vi "CTRE_Phoenix_MotorControl_PushMotionProfileTrajectory.vi"(0 "PhoenixMotorControlDevRef":T2={"DeviceStatus"={"status"=FALSE, "code"=0, "source"=""}, "Type"=enum."PWM", "PWM"={"PWM Channel"=enum."Invalid", "DeadBand"={"Name"="", "maxPositivePwm"=0, "minPositivePwm"=0, "centerPwm"=0, "maxNegativePwm"=0, "minNegativePwm"=0, "angularRange"=0}}, "CAN"={"Device Number"=0, "SetOutput VI Ref"=variant(enum8{"Percent VBus", "Current", "Speed", "Position", "Voltage"} enum."Percent VBus"), "GetOutput VI Ref"=variant(refnum<k1> refnum), "Enable VI Ref"=variant(dbl 12.0), "Disable VI Ref"=variant(enum8{"Percent VBus", "Speed", "Position", "Slave", "Unchanged / Invalid", "Voltage Compensation", "Current", "Motion Profile"} enum."Percent VBus"), "Data"=variant}, "Invert"=FALSE, "DIO PWM"={"PWM \"Enable\" Channel"=enum."Invalid", "DIOChannel"=enum."Invalid", "PWM Rate"=0.0}}, 1 "profileSlotSelect1":i32, 2 "durationMs":T1 items=["TrajectoryDuration_0ms"=0, "TrajectoryDuration_5ms"=5, "TrajectoryDuration_10ms"=10, "TrajectoryDuration_20ms"=20, "TrajectoryDuration_30ms"=30, "TrajectoryDuration_40ms"=40, "TrajectoryDuration_50ms"=50, "TrajectoryDuration_100ms"=100], 5 "position":dbl, 7 "velocity":dbl, 9 "auxiliaryPos":dbl, 11 "error in":errorcluster, 12 "profileSlotSelect0":i32, 13 "isLastPoint?":bool, 14 "Zero Position?":bool) -> (4 "PhoenixMotorControlDevRef":T2={"DeviceStatus"={"status"=FALSE, "code"=0, "source"=""}, "Type"=enum."PWM", "PWM"={"PWM Channel"=enum."Invalid", "DeadBand"={"Name"="", "maxPositivePwm"=0, "minPositivePwm"=0, "centerPwm"=0, "maxNegativePwm"=0, "minNegativePwm"=0, "angularRange"=0}}, "CAN"={"Device Number"=0, "SetOutput VI Ref"=variant(enum8{"Percent VBus", "Current", "Speed", "Position", "Voltage"} enum."Percent VBus"), "GetOutput VI Ref"=variant(refnum<k1> refnum), "Enable VI Ref"=variant(dbl 12.0), "Disable VI Ref"=variant(enum8{"Percent VBus", "Speed", "Position", "Slave", "Unchanged / Invalid", "Voltage Compensation", "Current", "Motion Profile"} enum."Percent VBus"), "Data"=variant}, "Invert"=FALSE, "DIO PWM"={"PWM \"Enable\" Channel"=enum."Invalid", "DIOChannel"=enum."Invalid", "PWM Rate"=0.0}}, 15 "error out":errorcluster)   [LabVIEW 2020]
doc: "Push another trajectory point into the top level buffer (which is emptied\ninto the motor controller's bottom buffer as room allows).\n\nThe members should be filled in with these values...\n\n <b>position</b> servo position in sensor units.\n <b> velocity</b> velocity to feed-forward in sensor units\n per 100ms.\n <b>headingDeg</b>\n <b>profileSlotSelect0</b> Which slot to get PIDF gains.\n PID is used for position servo.\n F is used as the Kv constant for velocity feed-forward.\n Typically this is hardcoded to the a particular slot, but you are free\n gain schedule if need be.\n Choose from [0,3].\n <b>profileSlotSelect1</b> Which slot to get PIDF gains for auxiliary PID.\n This only has impact during MotionProfileArc Control mode.\n Choose from [0,1].\n <b>isLastPoint</b> Set to true to signal Talon that this is the final point, so do not\n attempt to pop another trajectory point from out of the Talon buffer.\n Instead continue processing this way point. Typically the velocity\n member variable should be zero so that the motor doesn't spin indefinitely.\n <b>zeroPos</b> set to nonzero to signal motor controller to \"zero\" the selected\n position sensor before executing this trajectory point.\n Typically the first point should have this set only thus\n allowing the remainder of the MP positions to be relative to\n zero.\n <b>durationMs</b> Duration to apply this trajectory pt.\n This time unit is ADDED to the exising base time set by\n the ConfigMotionProfileTrajectoryPeriod VI."
uses:
  <vilib>/Rock Robotics/WPI/MotorControl/WPI_MotorControlDeviceRef.ctl
  <vilib>/Rock Robotics/WPI/MotorControl/WPI_MotorControlType.ctl
  <vilib>/Rock Robotics/SystemInterfaces/DIO/FPGA_DIOPWMChannel.ctl
  <vilib>/Rock Robotics/WPI/PWM/WPI_PWMDeadband.ctl
  <vilib>/Rock Robotics/SystemInterfaces/DIO/FPGA_DIOChannel.ctl
  <vilib>/Rock Robotics/WPI/ThirdParty/Phoenix-LabVIEW/Motor Controller/Controls/CTRE_Phoenix_MotorControl_TrajectoryPointTimeDur.ctl
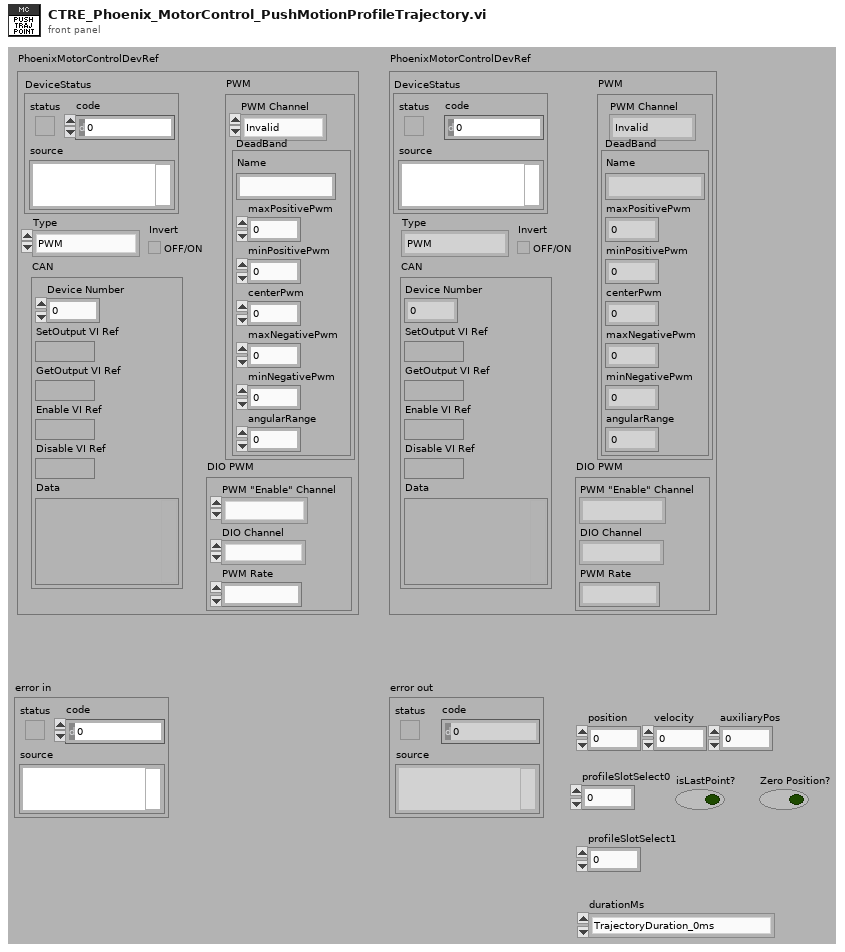
[diagram p1: front panel]
types:
  T1 = typedef "CTRE_Phoenix_MotorControl_TrajectoryPointTimeDur.ctl" = i32
  T2 = typedef "WPI_MotorControlDeviceRef.ctl" = cluster{"DeviceStatus":errorcluster, "Type":T3, "PWM":cluster{"PWM Channel":T4, "DeadBand":T5}, "CAN":cluster{"Device Number":u8, "SetOutput VI Ref":variant, "GetOutput VI Ref":variant, "Enable VI Ref":variant, "Disable VI Ref":variant, "Data":variant}, "Invert":bool, "DIO PWM":cluster{"PWM \"Enable\" Channel":T4, "DIOChannel":T6, "PWM Rate":dbl}}
  T3 = typedef "WPI_MotorControlType.ctl" = enum16{"PWM", "CAN", "DIO PWM"}
  T4 = typedef "FPGA_DIOPWMChannel.ctl" = enum8{"PWM 0", "PWM 1", "PWM 2", "PWM 3", "PWM 4", "PWM 5", "PWM 6", "PWM 7", "PWM 8", "PWM 9", "PWM MXP 0", "PWM MXP 1", "PWM MXP 2", "PWM MXP 3", "PWM MXP 4", "PWM MXP 5", "PWM MXP 6", "PWM MXP 7", "PWM MXP 8", "PWM MXP 9", "Invalid"}
  T5 = typedef "WPI_PWMDeadband.ctl" = cluster{"Name":string, "maxPositivePwm":i32, "minPositivePwm":i32, "centerPwm":i32, "maxNegativePwm":i32, "minNegativePwm":i32, "angularRange":u16}
  T6 = typedef "FPGA_DIOChannel.ctl" = enum8{"DIO 0", "DIO 1", "DIO 2", "DIO 3", "DIO 4", "DIO 5", "DIO 6", "DIO 7", "DIO 8", "DIO 9", "DIO MXP 0", "DIO MXP 1", "DIO MXP 2", "DIO MXP 3", "DIO MXP 4", "DIO MXP 5", "DIO MXP 6", "DIO MXP 7", "DIO MXP 8", "DIO MXP 9", "DIO MXP 10", "DIO MXP 11", "DIO MXP 12", "DIO MXP 13", "DIO MXP 14", "DIO MXP 15", "SPI Port CS1", "SPI Port CS2", "SPI Port CS3", "SPI Port MISO", "SPI Port MOSI", "Invalid"}
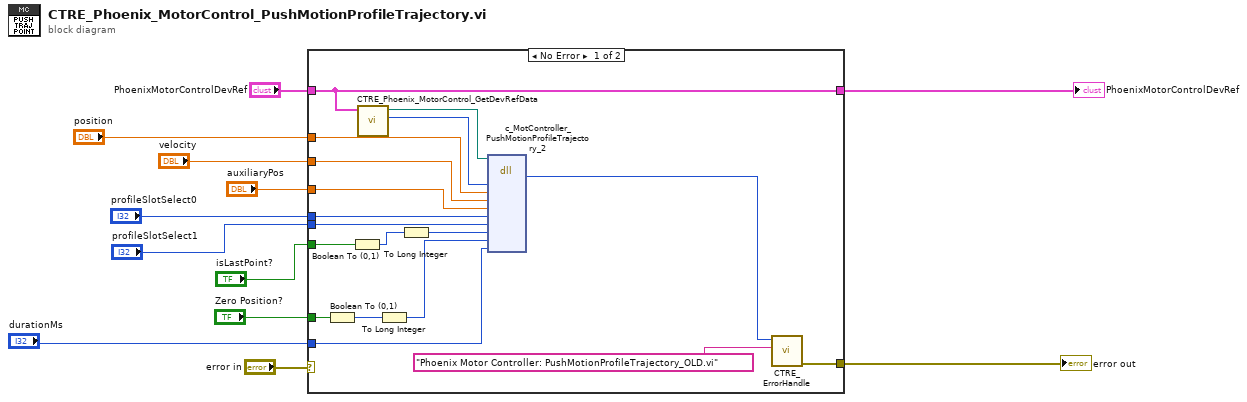
[diagram p0: block diagram]
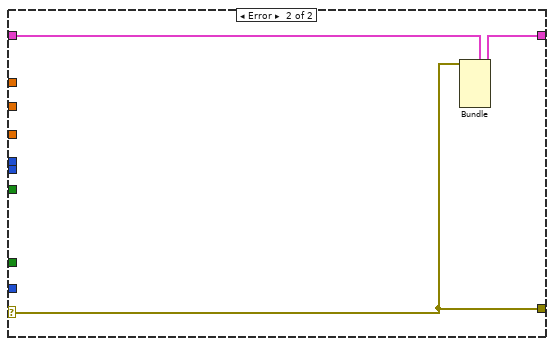
[diagram p2: hidden frame]
diagram:
  n1 = case shown="No Error" "error in" {
    selector: "error in" -> [_ w32]
    tunnel: "PhoenixMotorControlDevRef" -> [w30 w33]
    tunnel: [w27 w32] -> w11
    tunnel: [w30 w31] -> w9
    tunnel: "profileSlotSelect0" -> [w24 _]
    tunnel: "isLastPoint?" -> [w23 _]
    tunnel: "Zero Position?" -> [w21 _]
    tunnel: "position" -> [w17 _]
    tunnel: "velocity" -> [w16 _]
    tunnel: "auxiliaryPos" -> [w15 _]
    tunnel: "profileSlotSelect1" -> [w14 _]
    tunnel: "durationMs" -> [w13 _]
    frame No Error {
      n2 = Boolean To (0,1)(Boolean=w21) -> (0, 1=w20:i16)
      n3 = Boolean To (0,1)(Boolean=w23) -> (0, 1=w22:i16)
      n4 = call <vilib>:"CTRE_Phoenix_MotorControl_GetDevRefData.vi"("PhoenixMotorControlDevRef"=w30) -> ("handle"=w28:u64, "Library"=w29:path)  [unwired: 4 in, 5 out]
      n5 = To Long Integer(number=w20) -> (32bit integer=w18:i32)
      n6 = To Long Integer(number=w22) -> (32bit integer=w19:i32)
      n7 = dll-call lib="?" fn="c_MotController_PushMotionProfileTrajectory_2"(path in=w29, "handle"=w28, "position"=w17, "velocity"=w16, "headingDeg"=w15, "profileSlotSelect0"=w24, "profileSlotSelect1"=w14, "isLastPoint"=w19, "zeroPos"=w18, "durationMs"=w13) -> ("ErrorCode"=w26:i32)  [unwired: 11 in, 2 out]
      n8 = call <vilib>:"CTRE_ErrorHandle.vi"("origin"="Phoenix Motor Controller: PushMotionProfileTrajectory_OLD.vi", "code"=w26) -> ("error out"=w27:errorcluster)  [unwired: 9 in]
    }
    frame Error {
      n9 = Bundle(cluster=w33, "DeviceStatus"=w32) -> (w31:T2)  [unwired: 5 in]
    }
  }
  "PhoenixMotorControlDevRef" <- w9
  "error out" <- w11
